vi "Scan Setup.vi"(8 "error in (no error)":errorcluster, 11 "Two lockins reader in":refnum<class "Two lockins reader.lvclass">) -> (0 "error out":errorcluster, 3 "Two lockins reader out":refnum<class "Two lockins reader.lvclass">)   [LabVIEW 2017, in "Two lockins reader.lvclass"]
doc: "(Dynamic) Send commands to configure the instrument based on the class member fields."
uses:
  Two lockins reader.lvclass
  Reader/Reader.lvclass
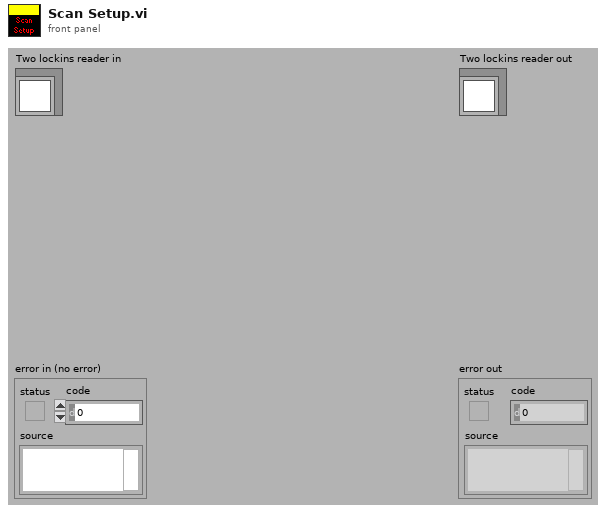
[diagram p1: front panel]
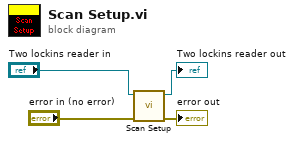
[diagram p0: block diagram]
diagram:
  n1 = call-parent "Scan Setup.vi"("error in (no error)"="error in (no error)", "Reader in"="Two lockins reader in") -> ("error out"=→"error out":errorcluster, "Reader out"=→"Two lockins reader out":refnum<class "Two lockins reader.lvclass">)  [unwired: 8 in]
